vi "20211224_03.vi"(1 "Side C":dbl caption="Side C(C邊)", 2 "Side B":dbl caption="Side B(B邊)", 3 "Angle A":dbl caption="Angle A(角度)") -> (0 "Area":dbl caption="Area(面積)")   [LabVIEW 2019]
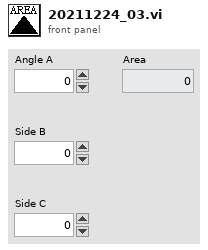
[diagram p1: front panel]
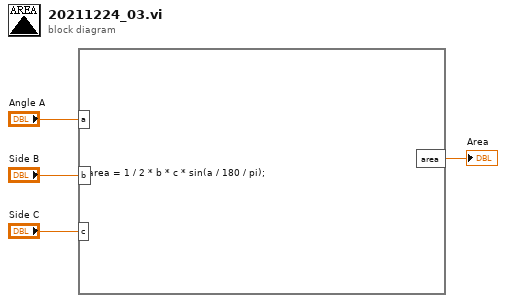
[diagram p0: block diagram]
diagram:
  n1 = formula code="area = 1 / 2 * b * c * sin(a / 180 / pi);"("a"="Angle A", "b"="Side B", "c"="Side C") -> ("area"=→"Area":dbl)
